vi "IMAQdx LL-Ring.vi"(8 "ErrIn":errorcluster, 11 "Camera":refnum<k21> caption="IMAQdx Session") -> (0 "ErrOut":errorcluster, 3 "ImgOut":T1[](array[typedef]))   [LabVIEW 2013]
doc: "Use this template to build a VI to use as a subVI."
uses:
  <vilib>/vision/Image Controls.llb/IMAQ Image.ctl
  <vilib>/vision/driver/IMAQdx.llb/IMAQdx Acquisition Mode.ctl
  <vilib>/vision/driver/IMAQdx.llb/IMAQdx Buffer Number Mode.ctl
  <vilib>/vision/driver/NI_Vision_Acquisition_Software.lvlib
panel:
  in  "stop":bool
  in  "Number of images":i32=10
  # "Input Parameters"
  # "Output Parameters"
  # "VI Description:\nLow Level IMAQ Sequence"
  # ":: MVI Framework V1.0 ::\nAuthor:Gaoke Yang\nEmail: gaoke.yang@yahoo.com\nWeb: www.mvicontrol.com\nCopyright (C) 2013, MVI Technologies All Rights Reserved"
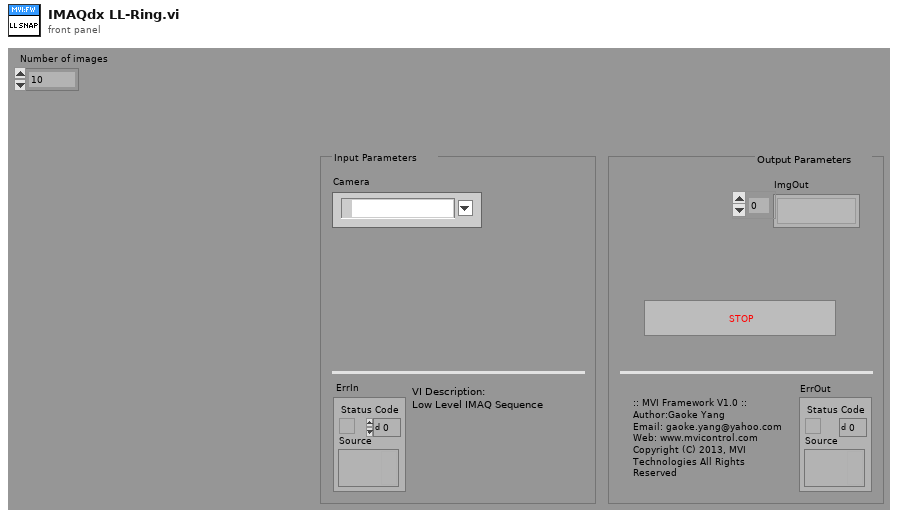
[diagram p1: front panel]
types:
  T1 = typedef "IMAQ Image.ctl" = refnum<image>
  T2 = typedef "NI_Vision_Acquisition_Software.lvlib/IMAQdx Buffer Number Mode.ctl" = enum32{"Next", "Last", "Buffer Number"}
  T3 = typedef "NI_Vision_Acquisition_Software.lvlib/IMAQdx Acquisition Mode.ctl" = enum32{"One Shot", "Continuous"}
  T4 = typedef "IMAQdx.ctl" = refnum<k21>
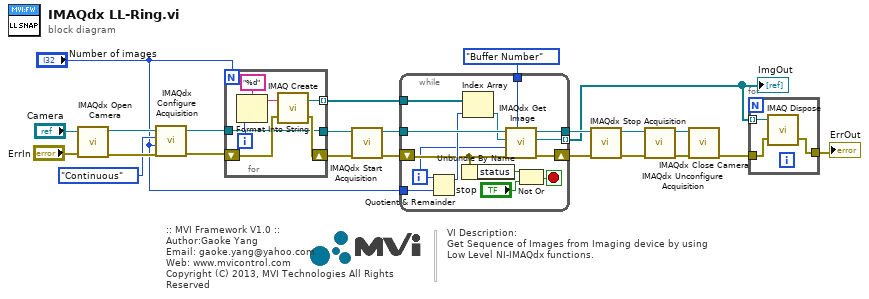
[diagram p0: block diagram]
diagram:
  # "VI Description:\nGet Sequence of Images from Imaging device by using \nLow Level NI-IMAQdx functions."
  # ":: MVI Framework V1.0 ::\nAuthor:Gaoke Yang\nEmail: gaoke.yang@yahoo.com\nWeb: www.mvicontrol.com\nCopyright (C) 2013, MVI Technologies All Rights Reserved"
  n1 = call <vilib>:"IMAQdx Open Camera.vi"("error in"="ErrIn", "Session In"="Camera") -> ("error out"=w20:errorcluster, "Session Out"=w19:T4)  [unwired: 8 in]
  n2 = call <vilib>:"IMAQdx Configure Acquisition.vi"("error in"=w20, "Number of Buffers"="Number of images", "Continuous?"=IMAQdx_Acquisition_Mode."Continuous", "Session In"=w19) -> ("error out"=w3:errorcluster, "Session Out"=w17:T4)  [unwired: 6 in]
  n3 = for {
    N: "Number of images" -> [_]
    shift-right: [w26] -> w15
    shift-left: w3 -> [w30]
    tunnel: [w25] -> w21 mode=indexing
    tunnel: w17 -> [w24]
    tunnel: [w24] -> w16
    i -> [w27]
    n4 = Format Into String(format string="%d", w27) -> (resulting string=w29:string)  [unwired: 2 in, 1 out]
    n5 = call "IMAQ Create"("Image Name"=w29, "error in (no error)"=w30) -> ("New Image"=w25:T1, "error out"=w26:errorcluster)  [unwired: 2 in, 1 out]
  }
  n6 = call <vilib>:"IMAQdx Start Acquisition.vi"("error in"=w15, "Session In"=w16) -> ("error out"=w14:errorcluster, "Session Out"=w13:T4)  [unwired: 8 in]
  n7 = while {
    tunnel: [w44] -> w7
    shift-right: [w43] -> w6
    shift-left: w14 -> [w33]
    tunnel: w21 -> [w39]
    tunnel: w13 -> [w42]
    tunnel: IMAQdx_Buffer_Number_Mode."Buffer Number" ("Buffer Number Mode (Next)") -> [w41]
    tunnel: [w40] -> w4 mode=indexing
    tunnel: "Number of images" -> [w36]
    i -> [w31]
    stop <- w32 stop-if-true
    n8 = Quotient & Remainder(x=w31, y=w36) -> (x-y*floor(x/y)=w38:i32)  [unwired: 1 out]
    n9 = Unbundle By Name(w33) -> ("status"=w35:bool)
    n10 = Index Array(array=w39, index=w38) -> (element=w37:T1)
    n11 = call <vilib>:"IMAQdx Get Image.vi"("Buffer Number Mode (Next)"=w41, "error in"=w33, "Buffer Number In"=w31, "Image In"=w37, "Session In"=w42) -> ("error out"=w43:errorcluster, "Image Out"=w40:T1, "Session Out"=w44:T4)  [unwired: 3 in, 1 out]
    n12 = Not Or(1:"stop", 2:w35) -> (0:w32:bool)
  }
  "ImgOut" <- w4
  n13 = call <vilib>:"IMAQdx Stop Acquisition.vi"("error in"=w6, "Session In"=w7) -> ("error out"=w10:errorcluster, "Session Out"=w11:T4)  [unwired: 8 out]
  n14 = call <vilib>:"IMAQdx Unconfigure Acquisition.vi"("error in"=w10, "Session In"=w11) -> ("error out"=w9:errorcluster, "Session Out"=w8:T4)  [unwired: 8 out]
  n15 = call <vilib>:"IMAQdx Close Camera.vi"("error in"=w9, "Session In"=w8) -> ("error out"=w5:errorcluster)  [unwired: 9 out]
  n16 = for {
    tunnel: w5 -> [w46]
    tunnel: w4 -> [w47] mode=indexing
    tunnel: [w45] -> w22
    n17 = call "IMAQ Dispose"("Image"=w47, "error in (no error)"=w46) -> ("error out"=w45:errorcluster)  [unwired: 1 in, 3 out]
  }
  "ErrOut" <- w22
